vi "Write JUnit Report.vi"(9 "Project Name":string, 10 "Test Results":refnum<class "Test Result.lvclass">[](array[class]), 11 "File Path":path) -> (0 "error out":errorcluster)   [LabVIEW 2017, in "Test Explorer.lvlib"]
uses:
  Test Explorer.lvlib
  Test Result/Test Result.lvclass
  <vilib>/ni/JUnit Results API/Controls/Test Suite Attribute Values.ctl
  Test Outcome.ctl
  Test Result/Test Result.lvclass/Test Result.ctl
  <vilib>/ni/JUnit Results API/Controls/Test Case Attributes.ctl
  Test Case/Test Case.lvclass/Test Case.ctl
  <vilib>/ni/JUnit Results API/Controls/Outcome Attributes.ctl
  Test Result/Get Outcome.vi
  Test Result/Get End Time.vi
  Test Result/Get Start Time.vi
  Test Result/Get Failure Message.vi
  Test Result/Get Test Case.vi
  Test Case/Get Qualified Name.vi
  Test Case/Test Case.lvclass
  <vilib>/ni/JUnit Results API/JUnit API.lvlib
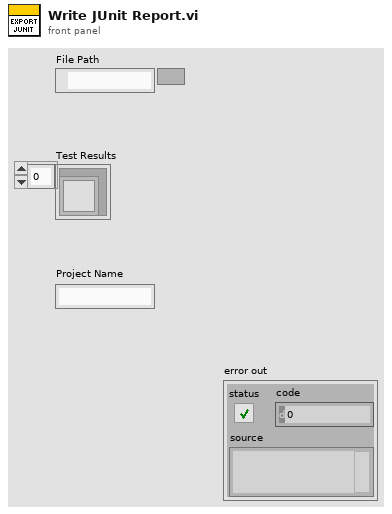
[diagram p1: front panel]
types:
  T1 = typedef "Test Outcome.ctl" = enum16{"None", "Passed", "Failed"}
  T2 = typedef "JUnit API.lvlib/Test Suite Attribute Values.ctl" = cluster{"name":string, "tests":i32, "failures":i32, "errors":i32, "time":dbl, "disabled":i32, "skipped":i32, "skips":i32, "timestamp":dbl, "hostname":string, "id":string, "package":string, "assertions":i32, "file":string, "skip":string, "log":string, "url":string}
  T3 = typedef "JUnit API.lvlib/Test Case Attributes.ctl" = cluster{"name":string, "assertions":i32, "time":dbl, "timestamp":dbl, "classname":string, "status":string, "class":string, "file":string, "line":string, "log":string, "group":string, "url":string}
  T4 = typedef "JUnit API.lvlib/Outcome Attributes.ctl" = cluster{"message":string, "type":string}
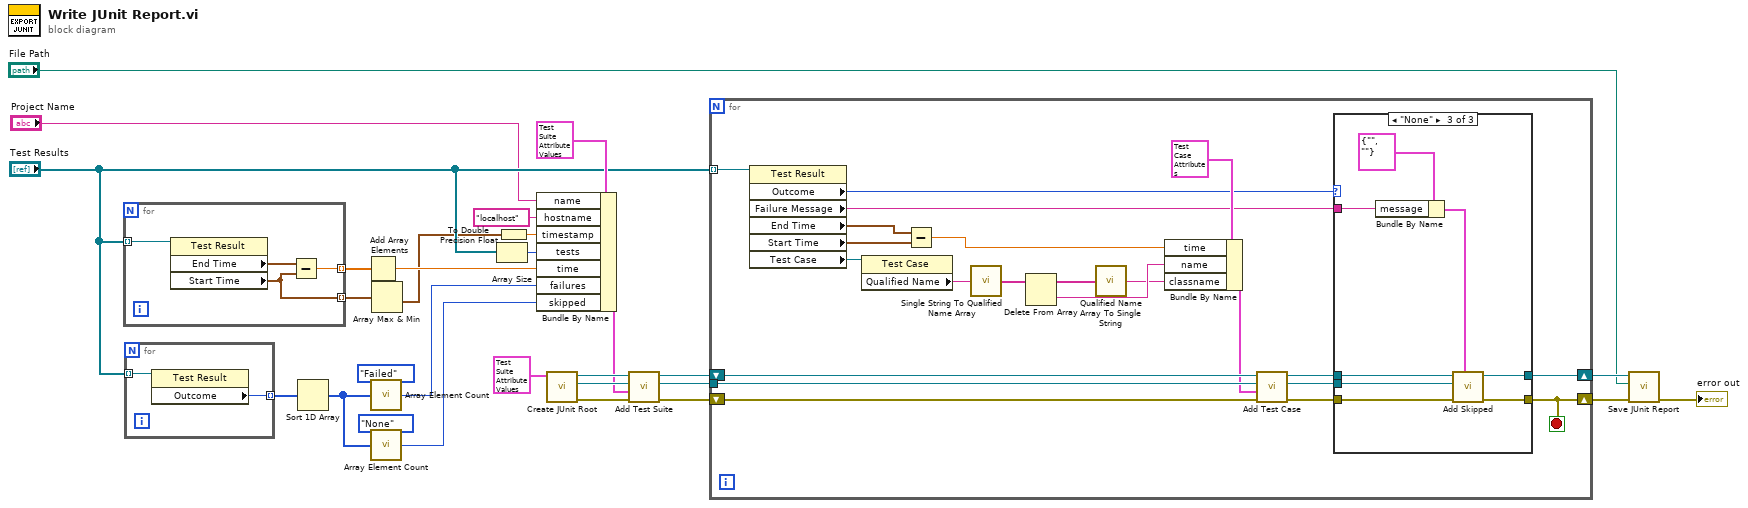
[diagram p0: block diagram]
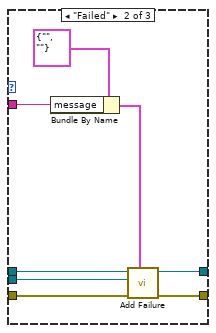
[diagram p3: hidden frame]
diagram:
  n1 = for {
    tunnel: "Test Results" -> [w32] mode=indexing
    tunnel: [w30] -> w18 mode=indexing
    tunnel: [w29] -> w4 mode=indexing
    n2 = property class="Test Result"(reference=w32) -> ("End Time"=w31:timestamp, "Start Time"=w29:timestamp)  [unwired: 1 in, 2 out]
    n3 = Subtract(x=w31, y=w29) -> (x-y=w30:dbl)
  }
  n4 = for {
    tunnel: "Test Results" -> [w34] mode=indexing
    tunnel: [w33] -> w13 mode=indexing
    n5 = property class="Test Result"(reference=w34) -> ("Outcome"=w33:T1)  [unwired: 1 in, 2 out]
  }
  n6 = Sort 1D Array(array=w13) -> (sorted array=w7:T1[])
  n7 = Add Array Elements(numeric array=w18) -> (sum=w17:dbl)
  n8 = call "Array Element Count.vi"("Array"=w7, "Element"=Test_Outcome."Failed" ("Outcome")) -> ("Count"=w9:i16)
  n9 = call "Array Element Count.vi"("Array"=w7, "Element"=Test_Outcome."None" ("Outcome")) -> ("Count"=w6:i16)
  n10 = Array Max & Min(array=w4) -> (min value=w3:timestamp)  [unwired: 3 out]
  n11 = Array Size(array="Test Results") -> (size(s)=w11:i32)
  n12 = To Double Precision Float(number=w3) -> (double precision float=w2:dbl)
  n13 = Bundle By Name(cluster=T2 {"name"="", "tests"=-1, "failures"=-1, "errors"=-1, "time"=-1.0, "disabled"=-1, "skipped"=-1, "skips"=-1, "timestamp"=-1.0, "hostname"="", "id"="", "package"="", "assertions"=-1, "file"="", "skip"="", "log"="", "url"=""} ("Test Suite Atrributes"), "name"="Project Name", "hostname"="localhost", "timestamp"=w2, "tests"=w11, "time"=w17, "failures"=w9, "skipped"=w6) -> (w14:T2)
  n14 = call <vilib>:"Create JUnit Root.vi"("Test Suites Atrributes"=T2 {"name"="", "tests"=-1, "failures"=-1, "errors"=-1, "time"=-1.0, "disabled"=-1, "skipped"=-1, "skips"=-1, "timestamp"=-1.0, "hostname"="", "id"="", "package"="", "assertions"=-1, "file"="", "skip"="", "log"="", "url"=""}) -> ("Error Out"=w25:errorcluster, "Teststuites Ref"=w23:refnum<k20>, "File Ref Out"=w28:refnum<k20>)  [unwired: 8 in]
  n15 = call <vilib>:"Add Test Suite.vi"("Error In (No Error)"=w25, "Test Suite Atrributes"=w14, "Teststuites Ref In"=w23, "File Ref In"=w28) -> ("Error Out"=w26:errorcluster, "Testsuite Ref"=w24:refnum<k20>, "File Ref Out"=w27:refnum<k20>)  [unwired: 4 in, 1 out]
  n16 = for {
    tunnel: w24 -> [w54]
    tunnel: "Test Results" -> [w48] mode=indexing
    shift-right: [w50] -> w21
    shift-left: w27 -> [w56]
    shift-right: [w49] -> w22
    shift-left: w26 -> [w55]
    stop <- w49 stop-if-true
    n17 = property class="Test Result"(reference=w48) -> ("Outcome"=w44:T1, "Failure Message"=w43:string, "End Time"=w41:timestamp, "Start Time"=w42:timestamp, "Test Case"=w46:refnum<class "Test Case.lvclass">)  [unwired: 1 in, 2 out]
    n18 = property class="Test Case"(reference=w46) -> ("Qualified Name"=w39:string)  [unwired: 1 in, 2 out]
    n19 = Subtract(x=w41, y=w42) -> (x-y=w40:dbl)
    n20 = call <vilib>:"Single String To Qualified Name Array.vi"("Fully Qualified String"=w39) -> ("Fully Qualified Array"=w38:string[])
    n21 = Delete From Array(array=w38) -> (deleted portion=w37:string, array with subset deleted=w36:string[])  [unwired: 2 in]
    n22 = call <vilib>:"Qualified Name Array To Single String.vi"("Fully Qualified Array"=w36) -> ("Fully Qualified String"=w35:string)
    n23 = Bundle By Name(cluster=T3 {"name"="", "assertions"=-1, "time"=-1.0, "timestamp"=-1.0, "classname"="", "status"="", "class"="", "file"="", "line"="", "log"="", "group"="", "url"=""} ("Test Case Atrributes"), "time"=w40, "name"=w37, "classname"=w35) -> (w45:T3)
    n24 = call <vilib>:"Add Test Case.vi"("Error In (No Error)"=w55, "Test Case Atrributes"=w45, "Testsuite Ref In"=w54, "File Ref In"=w56) -> ("error out"=w53:errorcluster, "Testcase Ref"=w52:refnum<k20>, "File Ref Out"=w51:refnum<k20>)  [unwired: 4 in, 1 out]
    n25 = case shown="\"None\"" w44 {
      tunnel: w53 -> [w57 w66 w74]
      tunnel: w52 -> [_ w65 w73]
      tunnel: w51 -> [w58 w64 w72]
      tunnel: [w58 w63 w71] -> w50
      tunnel: [w57 w62 w70] -> w49
      tunnel: w43 -> [_ w59 w67]
      frame Default {
      }
      frame "Failed" {
        n26 = Bundle By Name(cluster=T4 {"message"="", "type"=""} ("Outcome Attributes"), "message"=w59) -> (w60:T4)
        n27 = call <vilib>:"Add Failure.vi"("Outcome Attributes"=w60, "Error In (No Error)"=w66, "Testcase Ref"=w65, "File Ref In"=w64) -> ("Error Out"=w62:errorcluster, "File Ref Out"=w63:refnum<k20>)  [unwired: 5 in, 1 out]
      }
      frame "None" {
        n28 = Bundle By Name(cluster=T4 {"message"="", "type"=""} ("Outcome Attributes"), "message"=w67) -> (w68:T4)
        n29 = call <vilib>:"Add Skipped.vi"("Outcome Attributes"=w68, "Error In (No Error)"=w74, "Testcase Ref"=w73, "File Ref In"=w72) -> ("Error Out"=w70:errorcluster, "File Ref Out"=w71:refnum<k20>)  [unwired: 5 in, 1 out]
      }
    }
  }
  n30 = call <vilib>:"Save JUnit Report.vi"("Error In (No Error)"=w22, "XML file path"="File Path", "File Ref In"=w21) -> ("Error Out"=→"error out":errorcluster)  [unwired: 8 in]
